vi "Real World Corrdinates.vi"(4 "Transformation Matrix":T1, 6 "coordinates [pix]":cluster{"X":dbl, "Y":dbl} {"Y" format="%.2f"; "X" format="%.2f"}, 7 "FOV":cluster{"X [um]":dbl, "Y [um]":dbl} {"Y [um]" format="%.2f"; "X [um]" format="%.2f"}, 10 "Scope Position":T2, 11 "Image Area":cluster{"Width":u32, "Height":u32}) -> (1 "Target Coordinates":T2)   [LabVIEW 2012, in "Visual Analyser.lvlib"]
uses:
  Visual Analyser.lvlib
  <vilib>/Analysis/Matrix/Datatypes/RealMatrix.ctl
  <vilib>/Analysis/baseanly.llb/Real A x B.vi
  <vilib>/Analysis/NI_AALBase.lvlib
  <vilib>/Analysis/Matrix/NI_Matrix.lvlib
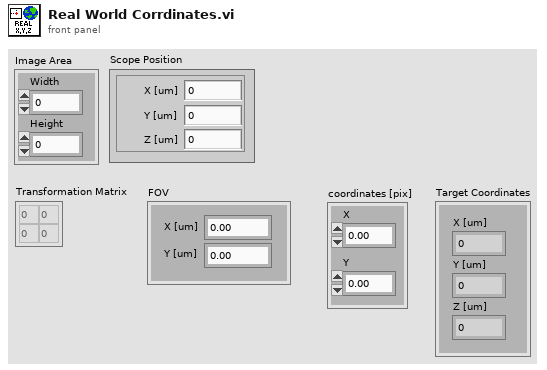
[diagram p1: front panel]
types:
  T1 = typedef "NI_Matrix.lvlib/RealMatrix.ctl" = dbl[][]
  T2 = cluster{"X [um]":dbl, "Y [um]":dbl, "Z [um]":dbl}
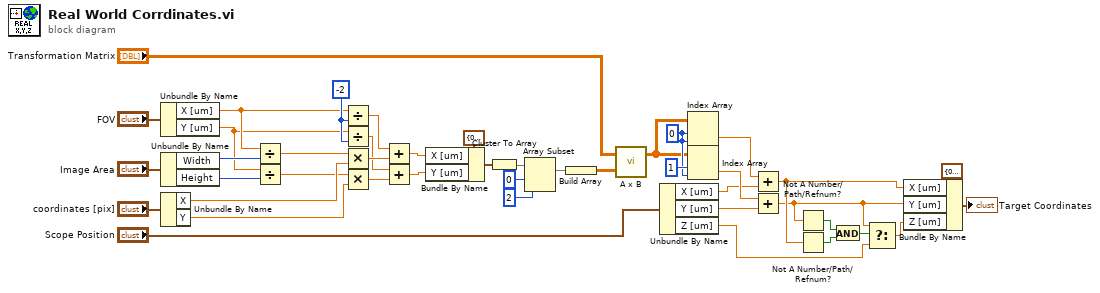
[diagram p0: block diagram]
diagram:
  w11 = -2 ("y")
  w33 = 0 ("index (row)")
  n1 = Unbundle By Name("FOV") -> ("X [um]"=w2:dbl, "Y [um]"=w1:dbl)
  n2 = Unbundle By Name("Image Area") -> ("Width"=w18:u32, "Height"=w19:u32)
  n3 = Unbundle By Name("coordinates [pix]") -> ("X"=w16:dbl, "Y"=w20:dbl)
  n4 = Divide(x=w2, y=w18) -> (x/y=w3:dbl)
  n5 = Divide(x=w1, y=w19) -> (x/y=w4:dbl)
  n6 = Divide(x=w2, y=w11) -> (x/y=w5:dbl)
  n7 = Divide(x=w1, y=w11) -> (x/y=w6:dbl)
  n8 = Multiply(x=w3, y=w16) -> (x*y=w7:dbl)
  n9 = Multiply(x=w4, y=w20) -> (x*y=w8:dbl)
  n10 = Add(x=w5, y=w7) -> (x+y=w9:dbl)
  n11 = Add(x=w6, y=w8) -> (x+y=w10:dbl)
  n12 = Bundle By Name(cluster=cluster{"X [um]":dbl, "Y [um]":dbl} {"X [um]"=0.0, "Y [um]"=0.0} ("input cluster"), "X [um]"=w9, "Y [um]"=w10) -> (w12:cluster{"X [um]":dbl, "Y [um]":dbl})
  n13 = Cluster To Array(cluster=w12) -> (array=w37:dbl[])
  n14 = Array Subset(array=w37, index=0, length=2) -> (w38:dbl[])
  n15 = Build Array(w38) -> (w40:T1)
  n16 = call-poly <vilib>:"A x B.vi"("B"=w40, "A"="Transformation Matrix") -> ("A x B"=w32:T1)  [unwired: 1 out]
  n17 = Unbundle By Name("Scope Position") -> ("X [um]"=w28:dbl, "Y [um]"=w31:dbl, "Z [um]"=w24:dbl)
  n18 = Index Array(array=w32, index (row)=w33, index (col)=w33) -> (element=w29:dbl)
  n19 = Index Array(array=w32, index (row)=1 ("index (col)"), index (col)=w33) -> (element=w30:dbl)
  n20 = Add ("Add.vi")(x=w29, y=w28) -> (x+y=w22:dbl)
  n21 = Add ("Add.vi")(x=w30, y=w31) -> (x+y=w21:dbl)
  n22 = Not A Number/Path/Refnum?(number/path/refnum=w21) -> (NaN/Path/Refnum?=w27:bool)
  n23 = Not A Number/Path/Refnum?(number/path/refnum=w22) -> (NaN/Path/Refnum?=w26:bool)
  n24 = And(x=w27, y=w26) -> (x .and. y?=w25:bool)
  n25 = Select(t=w21, s=w25, f=w24) -> (s? t:f=w23:dbl)
  n26 = Bundle By Name(cluster=T2 {"X [um]"=0.0, "Y [um]"=0.0, "Z [um]"=0.0} ("input cluster"), "X [um]"=w22, "Y [um]"=w21, "Z [um]"=w23) -> (→"Target Coordinates":T2)
